vi "Mini Bach random sampling_sub.vi"(2 "MNIST Input":dbl[][](array[numeric]), 3 "Mini Bach No.":i32) -> (0 "MNIST No.Row":dbl[](array[numeric]), 1 "MNIST Random Output":dbl[][](array[numeric]))   [LabVIEW 2021]
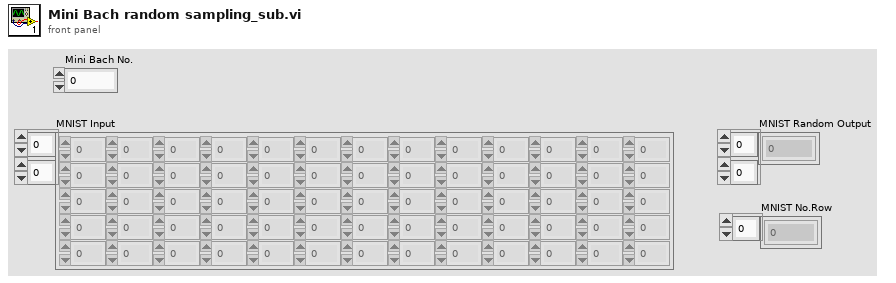
[diagram p1: front panel]
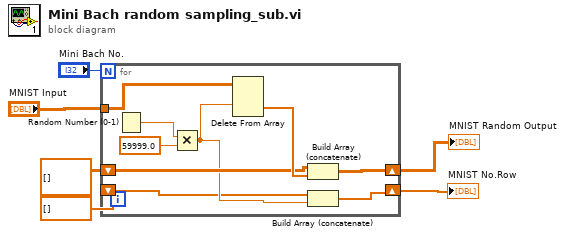
[diagram p0: block diagram]
diagram:
  n1 = for {
    N: "Mini Bach No." -> [_]
    shift-right: [w12] -> w5
    shift-left: dbl[][] [] -> [w11]
    shift-right: [w9] -> w4
    shift-left: dbl[] [] -> [w8]
    tunnel: "MNIST Input" -> [w7]
    n2 = Random Number (0-1)() -> (number: 0 to 1=w15:dbl)
    n3 = Multiply(x=w15, y=59999.0) -> (x*y=w10:dbl)
    n4 = Delete From Array(array=w7, index (row)=w10) -> (deleted portion=w13:dbl[])  [unwired: 2 in, 1 out]
    n5 = Build Array (concatenate)(w11, w13) -> (w12:dbl[][])
    n6 = Build Array (concatenate)(w8, w10) -> (w9:dbl[])
  }
  "MNIST Random Output" <- w5
  "MNIST No.Row" <- w4
